vi "UpdateStatus_SDG2.vi"(7 "error in":errorcluster, 10 "VISA resource":refnum<visa-resource-name>) -> (0 "error out":errorcluster)   [LabVIEW 2012]
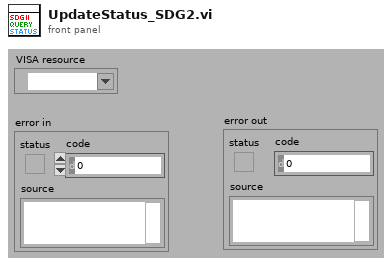
[diagram p1: front panel]
types:
  T1 = enum16{"Initialize", "Write", "Write/Read", "Read", "Clear", "Close"}
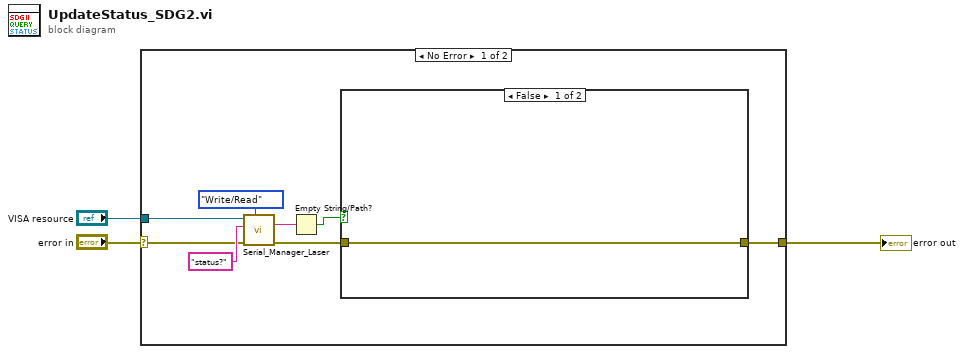
[diagram p0: block diagram]
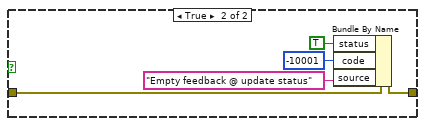
[diagram p2: hidden frame]
diagram:
  n1 = case shown="No Error" "error in" {
    selector: "error in" -> [w7 w18]
    tunnel: "VISA resource" -> [w10 _]
    tunnel: [w6 w18] -> w2
    frame No Error {
      n2 = call "Serial_Manager_Laser.vi"("Job"=T1."Write/Read", "error in"=w7, "write buffer"="status?", "VISA resource"=w10) -> ("error out"=w9:errorcluster, "read buffer"=w5:string)  [unwired: 6 in]
      n3 = Empty String/Path?(string/path=w5) -> (empty?=w4:bool)
      n4 = case shown="False" w4 {
        tunnel: w9 -> [w12 w17]
        tunnel: [w12 w16] -> w6
        frame False {
        }
        frame True {
          n5 = Bundle By Name(cluster=w17, "status"=TRUE, "code"=-10001, "source"="Empty feedback @ update status") -> (w16:errorcluster)
        }
      }
    }
    frame Error {
    }
  }
  "error out" <- w2
